vi "CalculateSSDArrays.vi"(10 "Template":u8[][](array[numeric]), 11 "Image":u8[][](array[numeric])) -> (3 "SSD":dbl[][](array[numeric]))   [LabVIEW 2014]
uses:
  LocalQuadraticSumArrays.vi
  FrequencyDomainCorrelationArrays.vi
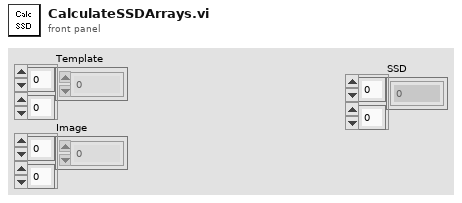
[diagram p1: front panel]
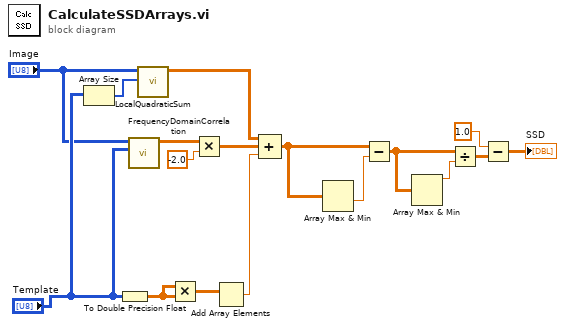
[diagram p0: block diagram]
diagram:
  n1 = Array Size(array="Template") -> (size(s)=w2:i32[])
  n2 = To Double Precision Float(number="Template") -> (double precision float=w6:dbl[][])
  n3 = call-poly "FrequencyDomainCorrelation.vi"("Template"="Template", "Image"="Image") -> ("FDCorrelation"=w4:dbl[][])  [unwired: 9 in]
  n4 = call-poly "LocalQuadraticSum.vi"("size(s)"=w2, "Image Pixels (U8)"="Image") -> ("localsum"=w1:dbl[][])  [unwired: 9 in]
  n5 = Multiply(x=w6, y=w6) -> (x*y=w16:dbl[][])
  n6 = Multiply(x=w4, y=-2.0) -> (x*y=w14:dbl[][])
  n7 = Add Array Elements(numeric array=w16) -> (sum=w15:dbl)
  n8 = Compound Arithmetic op=ADD(w1, w14, w15) -> (w13:dbl[][])
  n9 = Array Max & Min(array=w13) -> (min value=w12:dbl)  [unwired: 3 out]
  n10 = Subtract(x=w13, y=w12) -> (x-y=w9:dbl[][])
  n11 = Array Max & Min(array=w9) -> (max value=w10:dbl)  [unwired: 3 out]
  n12 = Divide(x=w9, y=w10) -> (x/y=w8:dbl[][])
  n13 = Subtract(x=1.0, y=w8) -> (x-y=→"SSD":dbl[][])
